vi "write_attributes.vi"(8 "error in (no error)":errorcluster, 10 "attributes":T1, 11 "GradientBoostingClassifier in":refnum<class "GradientBoostingClassifier.lvclass">) -> (0 "error out":errorcluster, 3 "GradientBoostingClassifier out":refnum<class "GradientBoostingClassifier.lvclass">)   [LabVIEW 2020, in "GradientBoostingClassifier.lvclass"]
uses:
  GradientBoostingClassifier.lvclass
  Controls/gradient_boosting_classifier_attributes.ctl
  GradientBoostingClassifier.lvclass/GradientBoostingClassifier.ctl
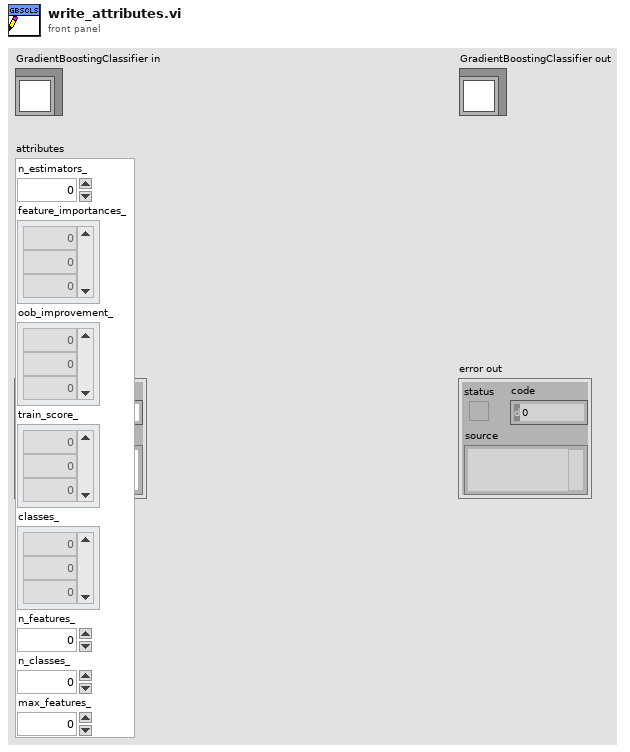
[diagram p1: front panel]
types:
  T1 = typedef "gradient_boosting_classifier_attributes.ctl" = cluster{"n_estimators_":dbl, "feature_importances_":dbl[], "oob_improvement_":dbl[], "train_score_":dbl[], "classes_":dbl[], "n_features_":dbl, "n_classes_":dbl, "max_features_":dbl}
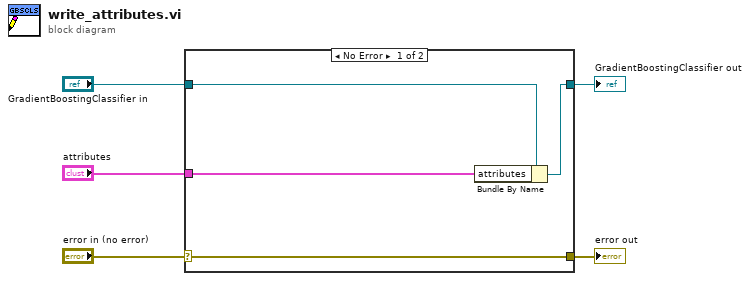
[diagram p0: block diagram]
diagram:
  n1 = case shown="No Error" "error in (no error)" {
    selector: "error in (no error)" -> [w9 w10]
    tunnel: [w9 w10] -> w4
    tunnel: [w7 w11] -> w2
    tunnel: "GradientBoostingClassifier in" -> [w8 w11]
    tunnel: "attributes" -> [w6 _]
    frame No Error {
      n2 = Bundle By Name(cluster=w8, "attributes"=w6) -> (w7:refnum<class "GradientBoostingClassifier.lvclass">)
    }
    frame Error {
    }
  }
  "error out" <- w4
  "GradientBoostingClassifier out" <- w2
